vi "Format_Table_Data.vi"(0 "Table In":T2=[["2966C", "02", "Var", "5/13/2020", "22:00:38", "1 3", "117", "A", "35.00", "0", "UP", "0.1", "", ""], ["2966C", "02", "Var", "5/13/2020", "22:00:38", "1 3", "118", "A", "35.00", "0", "UP", "0.1", "", ""], ["2966C", "02", "Var", "5/13/2020", "22:00:38", "1 3", "119", "A", "35.00", "0", "UP", "0.1", "", ""], ["2966C", "02", "Var", "5/13/2020", "22:00:39", "1 3", "122", "A", "35.00", "0", "UP", "0.1", "", ""], ["2966C", "02", "Var", "5/13/2020", "22:00:39", "1 3", "130", "A", "35.00", "0", "UP", "0.1", "", ""], ["2966C", "02", "Var", "5/13/2020", "22:00:39", "1 3", "131", "A", "35.00", "0", "UP", "0.1", "", ""], ["2966C", "02", "Var", "5/13/2020", "22:00:40", "1 3", "132", "A", "35.00", "0", "UP", "0.1", "", ""]], 1 "Measured Resistance (Ohms)":string="0", 2 "Path":path=path "C:/Sandbox/Git_Sandbox/Tools/MEMS Resistance Char/Output.csv", 3 "Set Chuck Position":string="0 1 13 ", 4 "Design Site Enum":T3(ring), 5 "error in (no error)":errorcluster, 7 "4-Wire Forced Current (A)":dbl, 8 "Actuation Cluster":T1={"VPU (V)"=0, "VPD (V)"=0, "Actuation Direction Enum"=enum."UP", "UP Act Forced Current (A)"=0.0, "DN Act Forced Current (A)"=0.0}, 9 "Run Info Cluster":T4={"Comment"="Init", "Package"="BC", "Wafer#"="04", "Lot#"="2966C"}) -> (14 "Table Out":T2=[["2966C", "02", "Var", "5/13/2020", "22:00:38", "1 3", "117", "A", "35.00", "0", "UP", "0.1", "", ""], ["2966C", "02", "Var", "5/13/2020", "22:00:38", "1 3", "118", "A", "35.00", "0", "UP", "0.1", "", ""], ["2966C", "02", "Var", "5/13/2020", "22:00:38", "1 3", "119", "A", "35.00", "0", "UP", "0.1", "", ""], ["2966C", "02", "Var", "5/13/2020", "22:00:39", "1 3", "122", "A", "35.00", "0", "UP", "0.1", "", ""], ["2966C", "02", "Var", "5/13/2020", "22:00:39", "1 3", "130", "A", "35.00", "0", "UP", "0.1", "", ""], ["2966C", "02", "Var", "5/13/2020", "22:00:39", "1 3", "131", "A", "35.00", "0", "UP", "0.1", "", ""], ["2966C", "02", "Var", "5/13/2020", "22:00:40", "1 3", "132", "A", "35.00", "0", "UP", "0.1", "", ""]], 19 "error out":errorcluster)   [LabVIEW 2017]
uses:
  Controls/Table.ctl
  <vilib>/Utility/file.llb/Write Delimited Spreadsheet (string).vi
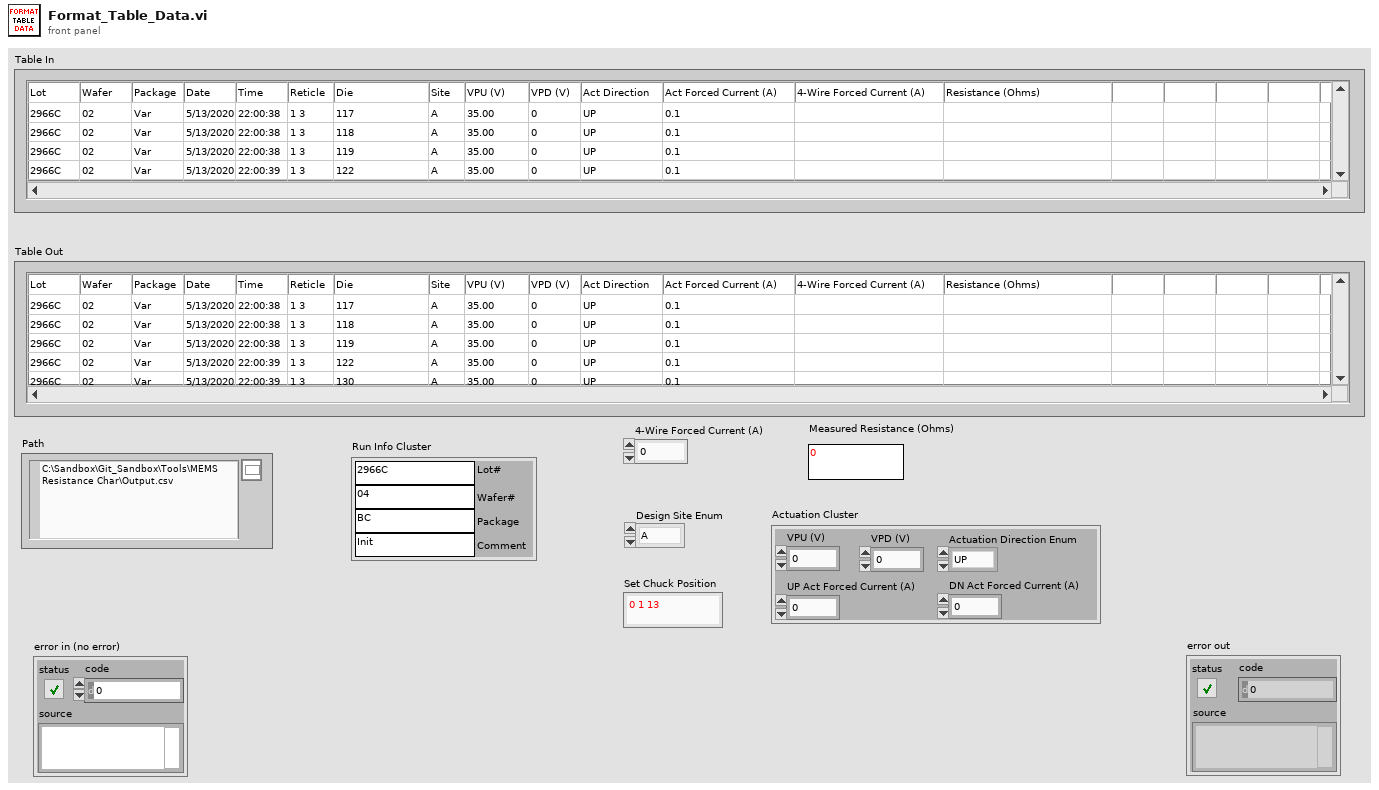
[diagram p1: front panel]
types:
  T1 = cluster{"VPU (V)":i64, "VPD (V)":i64, "Actuation Direction Enum":enum16{"DOWN", "UP"}, "UP Act Forced Current (A)":dbl, "DN Act Forced Current (A)":dbl}
  T2 = typedef "Table.ctl" = string[][]
  T3 = enum16{"A", "B", "C", "D", "E", "F", "G", "H", "I", "J"}
  T4 = cluster{"Comment":string, "Package":string, "Wafer#":string, "Lot#":string}
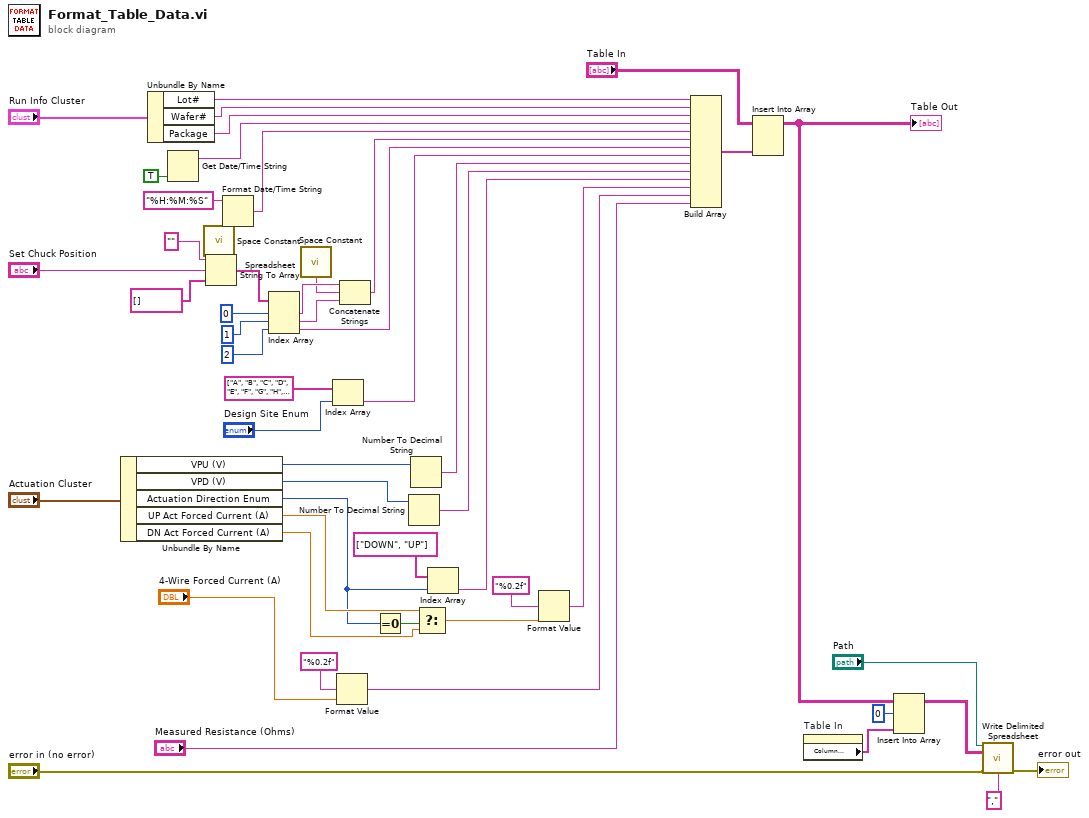
[diagram p0: block diagram]
diagram:
  n1 = Unbundle By Name("Actuation Cluster") -> ("VPU (V)"=w20:i64, "VPD (V)"=w19:i64, "Actuation Direction Enum"=w16:enum16{"DOWN", "UP"}, "UP Act Forced Current (A)"=w18:dbl, "DN Act Forced Current (A)"=w15:dbl)
  n2 = Unbundle By Name("Run Info Cluster") -> ("Lot#"=w36:string, "Wafer#"=w35:string, "Package"=w34:string)
  n3 = Get Date/Time String(want seconds? (F)=TRUE) -> (date string=w33:string)  [unwired: 2 in, 1 out]
  n4 = call <vilib>:"Space Constant.vi"() -> ("String"=w42:string)
  n5 = Spreadsheet String To Array(delimiter (Tab)=w42, format string="", spreadsheet string="Set Chuck Position", array type (2D Dbl)=string[] []) -> (array=w43:string[])
  n6 = Format Date/Time String(time format string (%c)="%H:%M:%S") -> (date/time string=w32:string)  [unwired: 2 in]
  n7 = Index Array(array=w43, index #1=0 ("index"), index #2=1 ("index"), index #3=2 ("index")) -> (element #1=w45:string, element #2=w46:string, element #3=w30:string)
  n8 = call <vilib>:"Space Constant.vi"() -> ("String"=w44:string)
  n9 = Index Array(array=string[] ["A", "B", "C", "D", "E", "F", "G", "H", "I", "J"], index="Design Site Enum") -> (element=w27:string)
  n10 = Format Value(format string="%0.2f", value (0)="4-Wire Forced Current (A)") -> (output string=w11:string)  [unwired: 1 in]
  n11 = Concatenate Strings(w45, w44, w46) -> (w31:string)
  n12 = Equal To 0?(x=w16) -> (x = 0?=w17:bool)
  n13 = Number To Decimal String(number=w19) -> (decimal integer string=w25:string)  [unwired: 1 in]
  n14 = Number To Decimal String(number=w20) -> (decimal integer string=w26:string)  [unwired: 1 in]
  n15 = Select(t=w18, s=w17, f=w15) -> (s? t:f=w13:dbl)
  n16 = Index Array(array=string[] ["DOWN", "UP"], index=w16) -> (element=w23:string)
  n17 = Format Value(format string="%0.2f", value (0)=w13) -> (output string=w12:string)  [unwired: 1 in]
  n18 = Build Array(w36, w35, w34, w33, w32, w31, w30, w27, w26, w25, w23, w12, w11, "Measured Resistance (Ohms)") -> (w8:string[])
  n19 = Insert Into Array(array="Table In", new element=w8) -> (w49:T2)  [unwired: 2 in]
  "Table Out" <- w49
  n20 = property on="Table In" class="Tbl (strict)"() -> ("Column Headers[]"=w5:string[])  [unwired: 2 in, 2 out]
  n21 = Insert Into Array(array=w49, index (row)=0, new element=w5) -> (w7:T2)  [unwired: 1 in]
  n22 = call-poly <vilib>:"Write Delimited Spreadsheet.vi"("file path (dialog if empty)"="Path", "2D data"=w7, "error in (no error)"="error in (no error)", "delimiter (\\t)"="," ("delimiter (\\t)")) -> ("error out"=→"error out":errorcluster)  [unwired: 10 in, 1 out]
